vi "Save_Params.vi"(1 "List In":string[](array[string]), 2 "Indicators":T1(array[cluster]), 3 "Controls":T1(array[cluster])) -> (0 "List Out":string[](array[string]))   [LabVIEW 2011]
panel:
  in  "Accept":bool
  in  "remove":bool
  in  "cancel":bool
  in  "Add":bool
  in  "Choix":u16(ring) items=["b", "y", "x", "z"]
  out "Strings Array":string[](array[string])
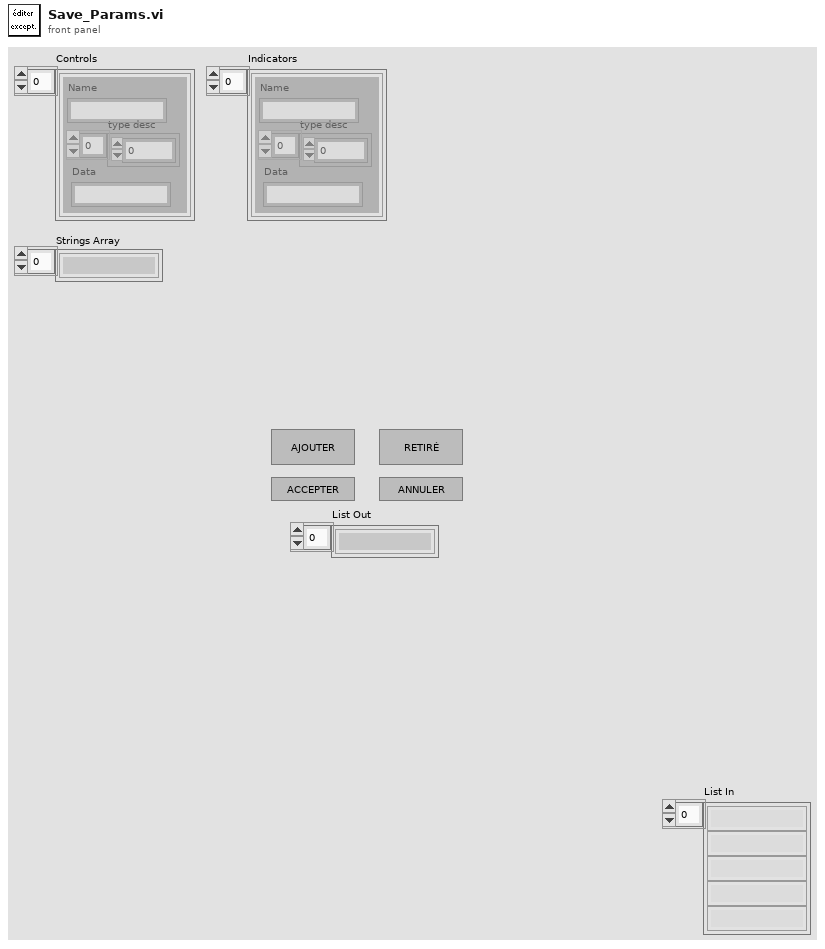
[diagram p1: front panel]
types:
  T1 = cluster{"Name":string, "type desc":i16[], "Data":string}[]
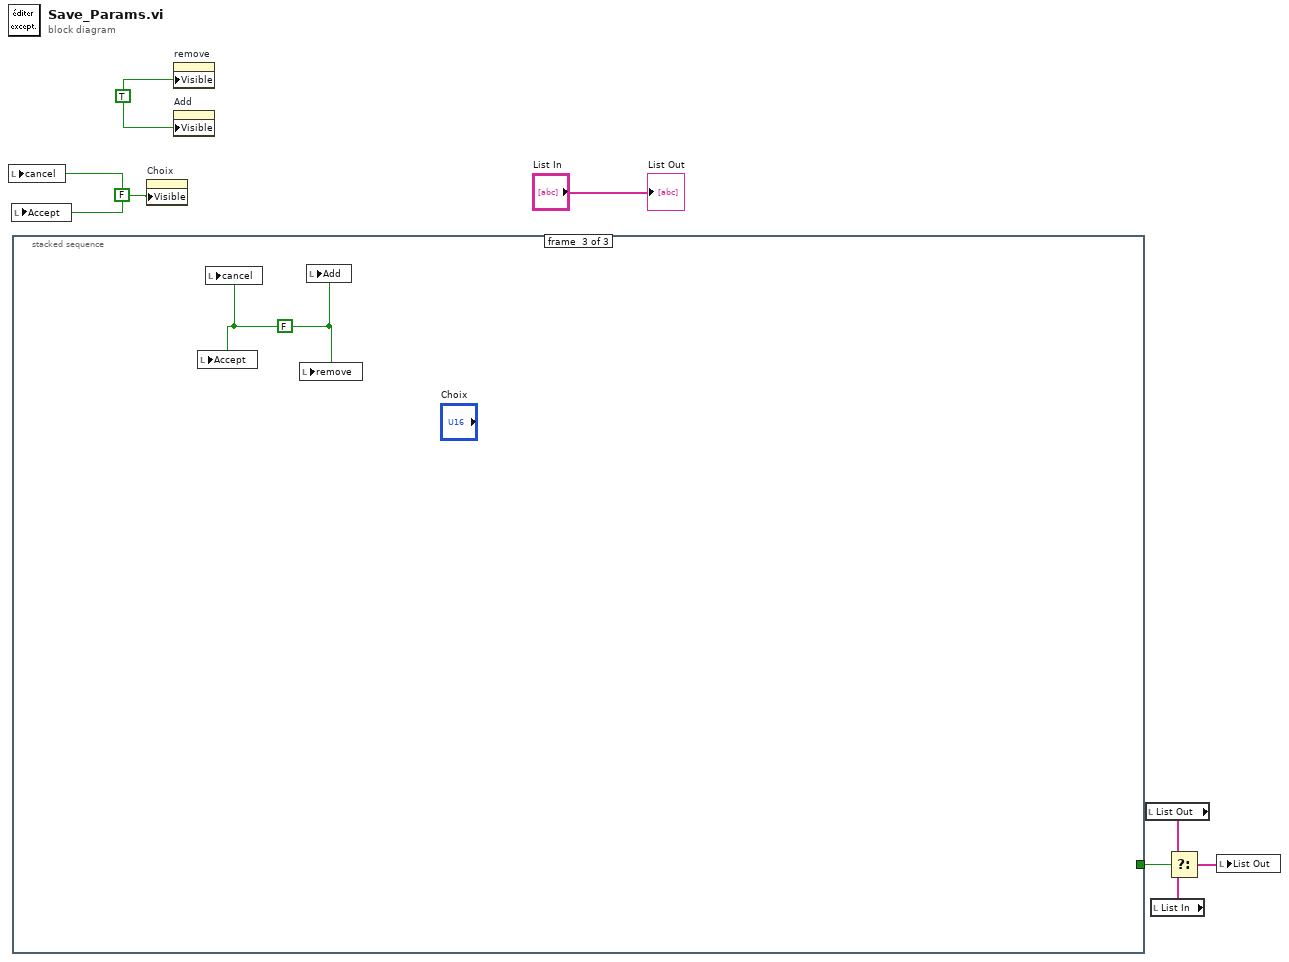
[diagram p0: block diagram]
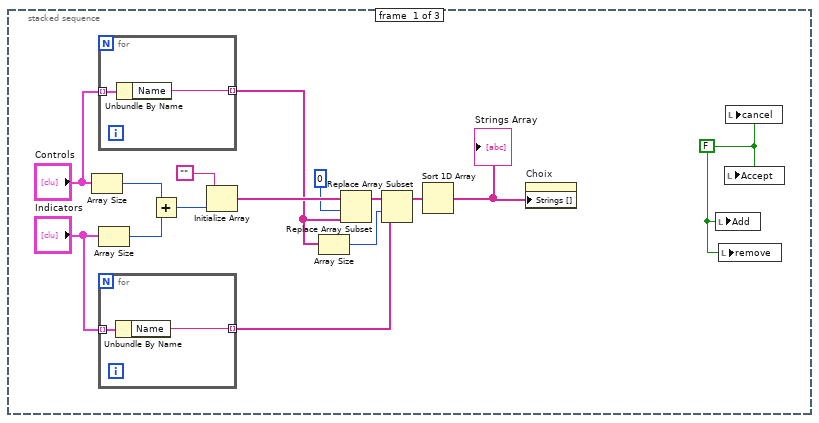
[diagram p2: hidden frame]
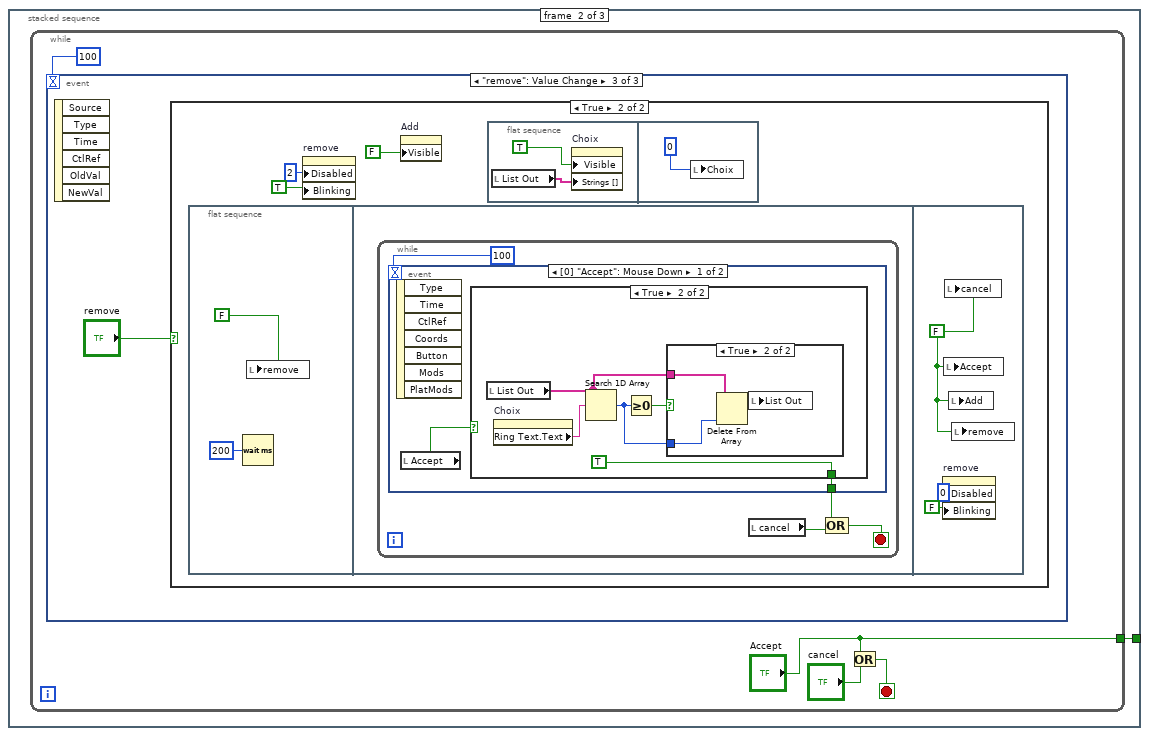
[diagram p3: hidden frame]
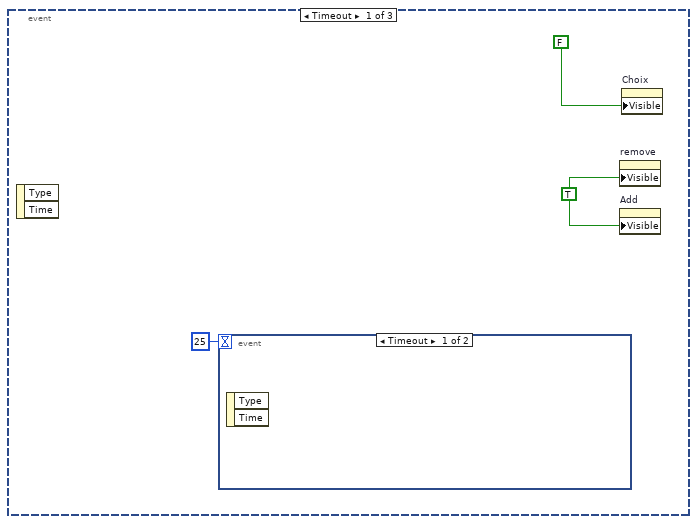
[diagram p4: hidden frame]
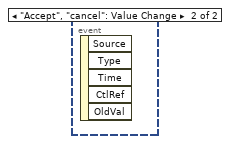
[diagram p5: hidden frame]
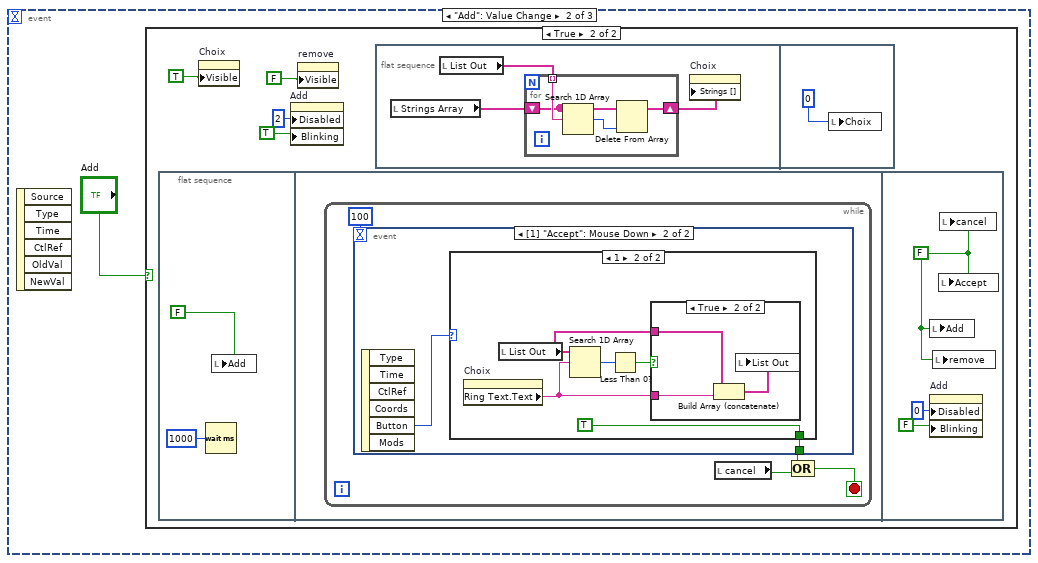
[diagram p6: hidden frame]
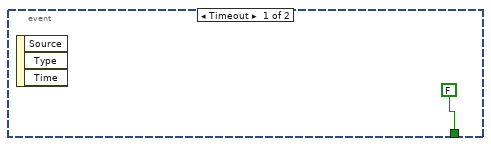
[diagram p8: hidden frame]
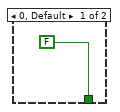
[diagram p9: hidden frame]
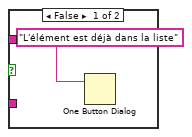
[diagram p10: hidden frame]
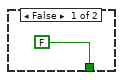
[diagram p12: hidden frame]
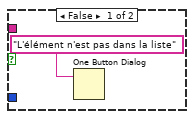
[diagram p13: hidden frame]
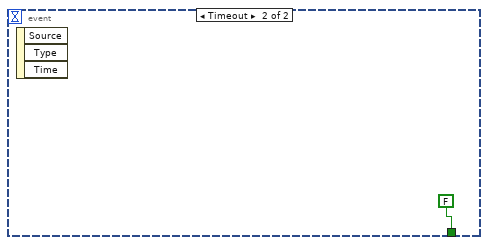
[diagram p14: hidden frame]
diagram:
  w1 = TRUE ("Visible")
  w2 = FALSE ("Visible")
  n1 = local write "cancel"(w2) -> ()
  n2 = local write "Accept"(w2) -> ()
  n3 = stacked-sequence {
    tunnel: [_ w27 _] -> w6
    frame #0 {
      w8 = FALSE
      n4 = Array Size(array="Controls") -> (size(s)=w22:i32)
      n5 = for {
        tunnel: "Controls" -> [w24] mode=indexing
        tunnel: [w23] -> w12 mode=indexing
        n6 = Unbundle By Name(w24) -> ("Name"=w23:string)
      }
      n7 = Array Size(array="Indicators") -> (size(s)=w21:i32)
      n8 = for {
        tunnel: "Indicators" -> [w26] mode=indexing
        tunnel: [w25] -> w10 mode=indexing
        n9 = Unbundle By Name(w26) -> ("Name"=w25:string)
      }
      n10 = Add(x=w22, y=w21) -> (x+y=w18:i32)
      n11 = Initialize Array("", w18) -> (w16:string[])
      n12 = Array Size(array=w12) -> (size(s)=w11:i32)
      n13 = Replace Array Subset(array=w16, new element=w12, index=0) -> (w14:string[])
      n14 = Replace Array Subset(array=w14, new element=w10, index=w11) -> (w13:string[])
      n15 = Sort 1D Array(array=w13) -> (sorted array=w9:string[])
      "Strings Array" <- w9
      n16 = property on="Choix" class="Ring (strict)"("Strings []"=w9) -> ()  [unwired: 2 in, 2 out]
      n17 = local write "Add"(w8) -> ()
      n18 = local write "remove"(w8) -> ()
      n19 = local write "Accept"(w8) -> ()
      n20 = local write "cancel"(w8) -> ()
    }
    frame #1 {
      n21 = while {
        tunnel: ["Accept"] -> w27
        stop <- w31 stop-if-true
        n22 = event shown="[2] \"remove\": Value Change" {
          selector: _ -> [_ _ _]
          dyn-events: _ -> [_ _ _]
          timeout: 100 -> [_ _ _]
          event Timeout {
            w33 = TRUE ("Visible")
            n23 = event-data() -> ()  [unwired: 1 in, 2 out]
            n24 = event shown="[0] Timeout" {
              selector: _ -> [_ _]
              dyn-events: _ -> [_ _]
              timeout: 25 -> [_ _]
              event Timeout {
                n25 = event-data() -> ()  [unwired: 1 in, 2 out]
              }
              event "Accept", "cancel": Value Change {
                n26 = event-data() -> ()  [unwired: 1 in, 5 out]
              }
            }
            n27 = property on="remove" class="Bool (strict)"("Visible"=w33) -> ()  [unwired: 2 in, 2 out]
            n28 = property on="Add" class="Bool (strict)"("Visible"=w33) -> ()  [unwired: 2 in, 2 out]
            n29 = property on="Choix" class="Ring (strict)"("Visible"=FALSE) -> ()  [unwired: 2 in, 2 out]
          }
          event "Add": Value Change {
            n30 = event-data() -> ()  [unwired: 1 in, 6 out]
            n31 = case shown="True" "Add" {
              frame False {
              }
              frame True {
                n32 = flat-sequence {
                  frame #0 {
                    n33 = Wait (ms)(milliseconds to wait=u32 1000) -> ()  [unwired: 1 out]
                    n34 = local write "Add"(FALSE) -> ()
                  }
                  frame #1 {
                    n35 = while {
                      stop <- w51 stop-if-true
                      n36 = event shown="[1] \"Accept\": Mouse Down" {
                        selector: _ -> [_ _]
                        dyn-events: _ -> [_ _]
                        timeout: 100 -> [_ _]
                        tunnel: [FALSE w55] -> w50
                        event Timeout {
                          n37 = event-data() -> ()  [unwired: 1 in, 3 out]
                        }
                        event "Accept": Mouse Down {
                          n38 = event-data() -> ("Button"=w56:u16)  [unwired: 1 in, 5 out]
                          n39 = case shown="1" w56 {
                            tunnel: [FALSE TRUE] -> w55
                            frame 0, Default {
                            }
                            frame 1 {
                              n40 = property on="Choix" class="Ring (strict)"() -> ("Ring Text.Text"=w61:string)  [unwired: 2 in, 2 out]
                              n41 = local read "List Out"() -> (w62:string[])
                              n42 = Search 1D Array(1D array=w62, element=w61) -> (index of element=w60:i32)  [unwired: 1 in]
                              n43 = Less Than 0?(x=w60) -> (x < 0?=w59:bool)
                              n44 = case shown="True" w59 {
                                tunnel: w62 -> [_ w65]
                                tunnel: w61 -> [_ w64]
                                frame False {
                                n45 = One Button Dialog(message="L'élément est déjà dans la liste") -> ()  [unwired: 1 in, 1 out]
                                }
                                frame True {
                                n46 = Build Array (concatenate)(w65, w64) -> (w66:string[])
                                n47 = local write "List Out"(w66) -> ()
                                }
                              }
                            }
                          }
                        }
                      }
                      n48 = local read "cancel"() -> (w52:bool)
                      n49 = Compound Arithmetic op=OR(w50, w52) -> (w51:bool)
                    }
                  }
                  frame #2 {
                    w67 = FALSE
                    n50 = local write "Add"(w67) -> ()
                    n51 = property on="Add" class="Bool (strict)"("Disabled"=u8 0, "Blinking"=FALSE) -> ()  [unwired: 2 in, 2 out]
                    n52 = local write "remove"(w67) -> ()
                    n53 = local write "Accept"(w67) -> ()
                    n54 = local write "cancel"(w67) -> ()
                  }
                }
                n55 = property on="Choix" class="Ring (strict)"("Visible"=TRUE) -> ()  [unwired: 2 in, 2 out]
                n56 = property on="Add" class="Bool (strict)"("Disabled"=u8 2, "Blinking"=TRUE) -> ()  [unwired: 2 in, 2 out]
                n57 = property on="remove" class="Bool (strict)"("Visible"=FALSE) -> ()  [unwired: 2 in, 2 out]
                n58 = flat-sequence {
                  frame #0 {
                    n59 = local read "Strings Array"() -> (w41:string[])
                    n60 = local read "List Out"() -> (w42:string[])
                    n61 = for {
                      tunnel: w42 -> [w46] mode=indexing
                      shift-right: [w44] -> w40
                      shift-left: w41 -> [w43]
                      n62 = Search 1D Array(1D array=w43, element=w46) -> (index of element=w45:i32)  [unwired: 1 in]
                      n63 = Delete From Array(array=w43, index=w45) -> (array with subset deleted=w44:string[])  [unwired: 1 in, 1 out]
                    }
                    n64 = property on="Choix" class="Ring (strict)"("Strings []"=w40) -> ()  [unwired: 2 in, 2 out]
                  }
                  frame #1 {
                    n65 = local write "Choix"(u16 0) -> ()
                  }
                }
              }
            }
          }
          event "remove": Value Change {
            n66 = event-data() -> ()  [unwired: 1 in, 6 out]
            n67 = case shown="True" "remove" {
              frame False {
              }
              frame True {
                n68 = flat-sequence {
                  frame #0 {
                    n69 = Wait (ms)(milliseconds to wait=u32 200) -> ()  [unwired: 1 out]
                    n70 = local write "remove"(FALSE ("Visible")) -> ()
                  }
                  frame #1 {
                    n71 = while {
                      stop <- w80 stop-if-true
                      n72 = event shown="[0] \"Accept\": Mouse Down" {
                        selector: _ -> [_ _]
                        dyn-events: _ -> [_ _]
                        timeout: 100 -> [_ _]
                        tunnel: [w84 FALSE] -> w79
                        event "Accept": Mouse Down {
                          n73 = event-data() -> ()  [unwired: 1 in, 7 out]
                          n74 = local read "Accept"() -> (w83:bool)
                          n75 = case shown="True" w83 {
                            tunnel: [FALSE TRUE] -> w84
                            frame False {
                            }
                            frame True {
                              n76 = local read "List Out"() -> (w90:string[])
                              n77 = property on="Choix" class="Ring (strict)"() -> ("Ring Text.Text"=w89:string)  [unwired: 2 in, 2 out]
                              n78 = Search 1D Array(1D array=w90, element=w89) -> (index of element=w87:i32)  [unwired: 1 in]
                              n79 = Greater Or Equal To 0?(x=w87) -> (x >= 0?=w88:bool)
                              n80 = case shown="True" w88 {
                                tunnel: w90 -> [_ w94]
                                tunnel: w87 -> [_ w92]
                                frame False {
                                n81 = One Button Dialog(message="L'élément n'est pas dans la liste") -> ()  [unwired: 1 in, 1 out]
                                }
                                frame True {
                                n82 = Delete From Array(array=w94, index=w92) -> (array with subset deleted=w93:string[])  [unwired: 1 in, 1 out]
                                n83 = local write "List Out"(w93) -> ()
                                }
                              }
                            }
                          }
                        }
                        event Timeout {
                          n84 = event-data() -> ()  [unwired: 1 in, 3 out]
                        }
                      }
                      n85 = local read "cancel"() -> (w81:bool)
                      n86 = Compound Arithmetic op=OR(w79, w81) -> (w80:bool)
                    }
                  }
                  frame #2 {
                    w96 = FALSE
                    n87 = property on="remove" class="Bool (strict)"("Disabled"=u8 0, "Blinking"=FALSE) -> ()  [unwired: 2 in, 2 out]
                    n88 = local write "Accept"(w96) -> ()
                    n89 = local write "cancel"(w96) -> ()
                    n90 = local write "Add"(w96) -> ()
                    n91 = local write "remove"(w96) -> ()
                  }
                }
                n92 = property on="remove" class="Bool (strict)"("Disabled"=u8 2, "Blinking"=TRUE) -> ()  [unwired: 2 in, 2 out]
                n93 = property on="Add" class="Bool (strict)"("Visible"=FALSE) -> ()  [unwired: 2 in, 2 out]
                n94 = flat-sequence {
                  frame #0 {
                    n95 = local read "List Out"() -> (w74:string[])
                    n96 = property on="Choix" class="Ring (strict)"("Visible"=TRUE, "Strings []"=w74) -> ()  [unwired: 2 in, 2 out]
                  }
                  frame #1 {
                    n97 = local write "Choix"(u16 0) -> ()
                  }
                }
              }
            }
          }
        }
        n98 = Or(x="Accept", y="cancel") -> (x .or. y?=w31:bool)
      }
    }
    frame #2 {
      w99 = FALSE ("Visible")
      n99 = local write "Accept"(w99) -> ()
      n100 = local write "cancel"(w99) -> ()
      n101 = local write "remove"(w99) -> ()
      n102 = local write "Add"(w99) -> ()
    }
  }
  n103 = property on="Choix" class="Ring (strict)"("Visible"=w2) -> ()  [unwired: 2 in, 2 out]
  n104 = property on="remove" class="Bool (strict)"("Visible"=w1) -> ()  [unwired: 2 in, 2 out]
  n105 = property on="Add" class="Bool (strict)"("Visible"=w1) -> ()  [unwired: 2 in, 2 out]
  n106 = local read "List Out"() -> (w4:string[])
  n107 = local read "List In"() -> (w3:string[])
  n108 = Select(t=w4, s=w6, f=w3) -> (s? t:f=w5:string[])
  n109 = local write "List Out"(w5) -> ()
  "List Out" <- "List In"
